vi "_Send Command.vi"(8 "error in (no error)":errorcluster, 9 "Read Value? (F)":bool, 10 "Command":string, 11 "VISA resource name":refnum<visa-resource-name>) -> (0 "error out":errorcluster, 2 "Response":string, 3 "VISA resource name out":refnum<visa-resource-name>)   [LabVIEW 2015, in "SRS SR400.lvlib"]
doc: "Writes the Command string to the device. If Read Value? is false, no return value is expected. If Read Value? is true, the command is a query, and the value associated with the Command is returned on the Response output terminal."
uses:
  SRS SR400.lvlib
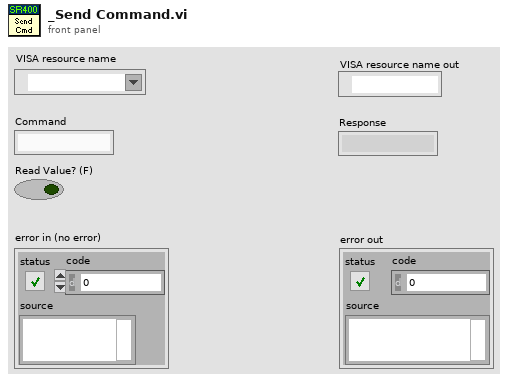
[diagram p1: front panel]
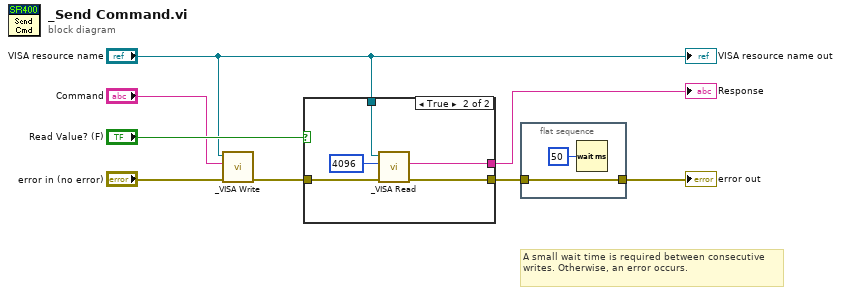
[diagram p0: block diagram]
diagram:
  # "A small wait time is required between consecutive writes. Otherwise, an error occurs."
  n1 = call "_VISA Write.vi"("error in (no error)"="error in (no error)", "Command"="Command", "VISA resource name"="VISA resource name") -> ("error out"=w6:errorcluster)  [unwired: 8 out]
  n2 = case shown="True" "Read Value? (F)" {
    tunnel: [_ w14] -> w5
    tunnel: w6 -> [w9 w13]
    tunnel: [w9 w12] -> w2
    tunnel: "VISA resource name" -> [_ w11]
    frame False {
    }
    frame True {
      n3 = call "_VISA Read.vi"("error in (no error)"=w13, "Byte Count"=u32 4096 ("byte count"), "VISA resource name"=w11) -> ("error out"=w12:errorcluster, "Response"=w14:string)  [unwired: 7 out]
    }
  }
  "Response" <- w5
  n4 = flat-sequence {
    tunnel: [w16] -> w1
    tunnel: w2 -> [w16]
    frame #0 {
      n5 = Wait (ms)(milliseconds to wait=u32 50) -> ()  [unwired: 1 out]
    }
  }
  "VISA resource name out" <- "VISA resource name"
  "error out" <- w1
